vi "题目五.vi"() -> ()   [LabVIEW 2017]
panel:
  out "平均数":dbl
  out "最小值":dbl
  out "最大值":dbl
  out "波形图":dbl[](graph)
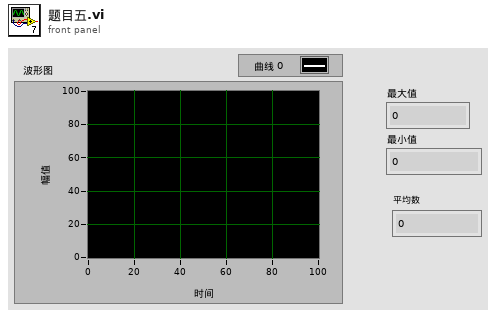
[diagram p1: front panel]
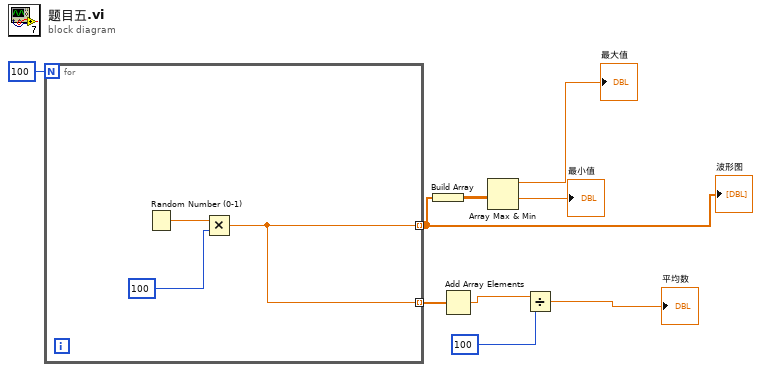
[diagram p0: block diagram]
diagram:
  n1 = for {
    N: 100 -> [_]
    tunnel: [w10] -> w4 mode=indexing
    tunnel: [w10] -> w1 mode=indexing
    n2 = Random Number (0-1)() -> (number: 0 to 1=w12:dbl)
    n3 = Multiply(x=w12, y=100) -> (x*y=w10:dbl)
  }
  "波形图" <- w4
  n4 = Build Array(w4) -> (w8:dbl[][])
  n5 = Add Array Elements(numeric array=w1) -> (sum=w2:dbl)
  n6 = Array Max & Min(array=w8) -> (max value=→"最大值":dbl, min value=→"最小值":dbl)  [unwired: 2 out]
  n7 = Divide(x=w2, y=100) -> (x/y=→"平均数":dbl)
